vi "Set Initialization Data - Modbus PLC 2.vi"(8 "error in":errorcluster, 11 "gui in":refnum<class "gui.lvclass">) -> (0 "error out":errorcluster, 3 "gui out":refnum<class "gui.lvclass">)   [LabVIEW 2023, in "GUI.lvlib" / "gui.lvclass"]
doc: "In this VI you can set the initialization data of a statically-linked subWorker."
uses:
  gui.lvclass
  gui.lvclass/gui.ctl
  Modbus PLC/Modbus PLC/Response Cases.ctl
  Modbus PLC/Modbus PLC/Modbus PLC.lvclass
  Modbus PLC/Modbus PLC/Initialization Data.ctl
  J:/Work/Cortech/KTM 1001/Workers Hardware/Workers/Base Classes/Base Hardware/Base Hardware.lvclass
  C:/Program Files/National Instruments/LabVIEW 2023/vi.lib/addons/_Workers/Library/Classes/Worker/Worker.lvclass
  C:/Program Files/National Instruments/LabVIEW 2023/vi.lib/addons/_Workers/Library/Classes/Workers Object/Workers Object.lvclass
  J:/Work/Cortech/KTM 1001/Workers Hardware/Hardware Interface/Hardware Interface.lvclass
  J:/Work/Cortech/KTM 1001/Modbus PLC/Modbus PLC/Modbus PLC.lvclass
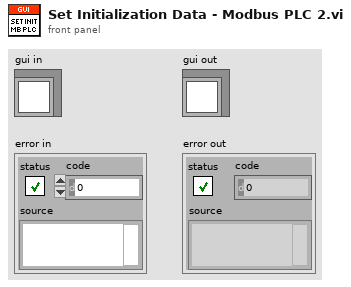
[diagram p1: front panel]
types:
  T1 = typedef "Modbus PLC.lvlib/Modbus PLC.lvclass/Initialization Data.ctl" = cluster{"Response Cases":T2}
  T2 = typedef "Modbus PLC.lvlib/Modbus PLC.lvclass/Response Cases.ctl" = cluster{"Placeholder - Can be deleted":string}
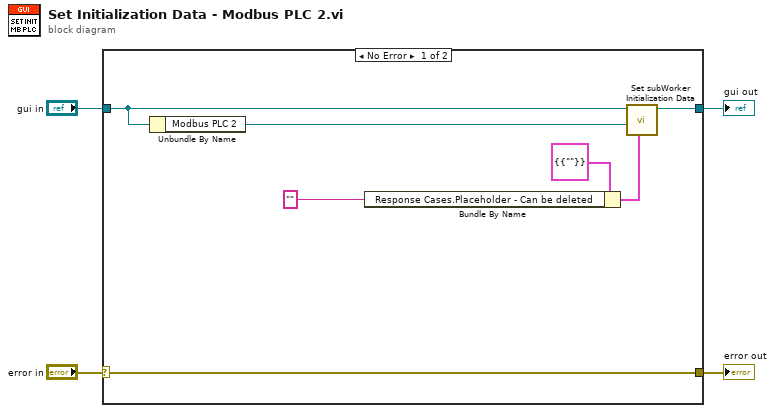
[diagram p0: block diagram]
diagram:
  n1 = case shown="No Error" "error in" {
    selector: "error in" -> [w11 w13]
    tunnel: [w11 w13] -> w3
    tunnel: [w9 w12] -> w2
    tunnel: "gui in" -> [w8 w12]
    frame No Error {
      n2 = Unbundle By Name(w8) -> ("Modbus PLC 2"=w10:refnum<class "Modbus PLC.lvclass">)
      n3 = Bundle By Name(cluster=T1 {"Response Cases"={"Placeholder - Can be deleted"=""}} ("Initialization Data"), "Response Cases.Placeholder - Can be deleted"="" ("Placeholder")) -> (w6:T1)
      n4 = call-dynamic "Set subWorker Initialization Data.vi"("Initialization Data"=w6, "subWorker"=w10, "Worker"=w8) -> ("Worker out"=w9:refnum<class "gui.lvclass">)  [unwired: 8 in]
    }
    frame Error {
    }
  }
  "error out" <- w3
  "gui out" <- w2
